vi "Save to file.vi"(8 "error in (no error)":errorcluster, 10 "Sent By":string, 11 "Log in":refnum<class "Log.lvclass">) -> (0 "error out":errorcluster)   [LabVIEW 2020, in "Log.lvlib" / "Log.lvclass"]
uses:
  Log.lvclass
  <vilib>/Utility/sysdir.llb/System Directory Type.ctl
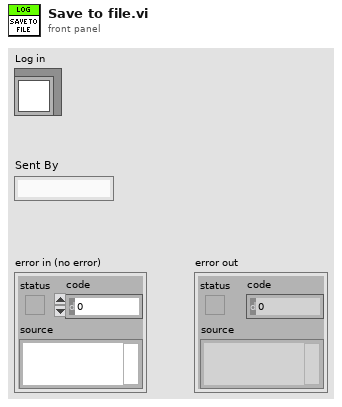
[diagram p1: front panel]
types:
  T1 = enum16{"open", "replace", "create", "open or create", "replace or create", "replace or create with confirmation"}
  T2 = typedef "System Directory Type.ctl" = i32
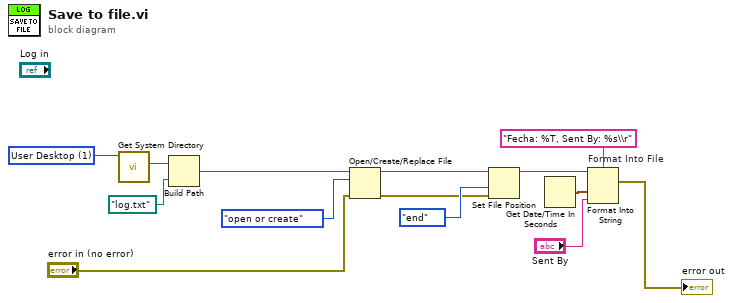
[diagram p0: block diagram]
diagram:
  w11 = T2 1 items=["User Home"=0, "User Desktop"=1, "User Documents"=2, "User Application Data"=3, "User Preferences"=4, "User Temporary"=5, "Public Documents"=6, "Public Application Data"=7, "Public Preferences"=8, "Public Cache"=13, "System Core Libraries"=9, "System Installed Libraries"=10, "Application Files"=11, "Boot Volume Root"=12] ("system directory type")
  n1 = call <vilib>:"Get System Directory.vi"("system directory type"=w11) -> ("system directory"=w10:path)  [unwired: 10 in]
  n2 = Build Path(base path=w10, name or relative path=path "log.txt") -> (appended path=w6:path)
  n3 = Open/Create/Replace File(file path (use dialog)=w6, error in="error in (no error)", operation (0:open)=T1."open or create") -> (refnum out=w4:refnum<file>, error out=w3:errorcluster)  [unwired: 3 in, 1 out]
  n4 = Set File Position(refnum=w4, from (0:start)=enum16{"start", "end", "current"}."end", error in=w3) -> (refnum out=w2:refnum<file>)  [unwired: 1 in, 1 out]
  n5 = Get Date/Time In Seconds() -> (seconds since 1Jan1904=w13:timestamp)
  n6 = Format Into String "Format Into File"(format string="Fecha: %T, Sent By: %s\\r", initial string=w2, w13, "Sent By") -> (error out=→"error out":errorcluster)  [unwired: 1 in, 1 out]
